vi "PDC_GetPartitionList.vi"(0 "DeviceNo":u32, 5 "ChildNo":u32, 11 "error in (no error)":errorcluster) -> (4 "ReturnValue":u32, 6 "Count":u32, 8 "Frames":u32[](array[numeric]), 10 "Blocks":u32[](array[numeric]), 14 "ErrorCode":u32, 15 "error out":errorcluster)   [LabVIEW 2015]
doc: "This VI retrieves the partition list of the specified child device."
uses:
  sub/global.vi
  PDCLIB.dll
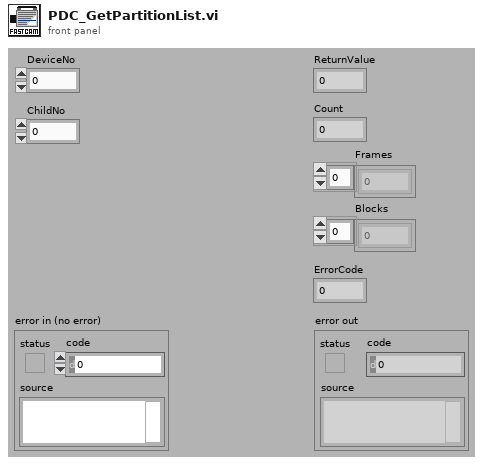
[diagram p1: front panel]
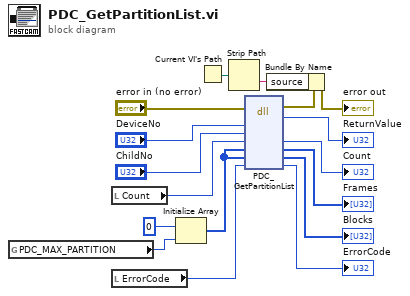
[diagram p0: block diagram]
diagram:
  n1 = global read "global.vi" "PDC_MAX_PARTITION"() -> (w10:i32)
  n2 = local read "Count"() -> (w11:u32)
  n3 = local read "ErrorCode"() -> (w14:u32)
  n4 = Initialize Array(u32 0, w10) -> (w6:u32[])
  n5 = Current VI's Path() -> (path=w3:path)
  n6 = Strip Path(path=w3) -> (name=w4:string)  [unwired: 1 out]
  n7 = dll-call lib="PDCLIB.dll" fn="PDC_GetPartitionList"(error in="error in (no error)", "nDeviceNo"="DeviceNo", "nChildNo"="ChildNo", "pCount"=w11, "pFrames"=w6, "pBlocks"=w6, "pErrorCode"=w14) -> (error out=w2:errorcluster, "return type"=→"ReturnValue":u32, "pCount"=→"Count":u32, "pFrames"=→"Frames":u32[], "pBlocks"=→"Blocks":u32[], "pErrorCode"=→"ErrorCode":u32)  [unwired: 4 in, 1 out]
  n8 = Bundle By Name(cluster=w2, "source"=w4) -> (→"error out":errorcluster)
